vi "Replace a Substring.vi"() -> ()   [LabVIEW 2016]
panel:
  out "Replaced Sub-String":string
  out "Result String":string
  in  "Offset":dbl
  in  "Sub-String":string
  in  "String":string
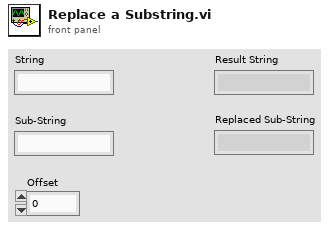
[diagram p1: front panel]
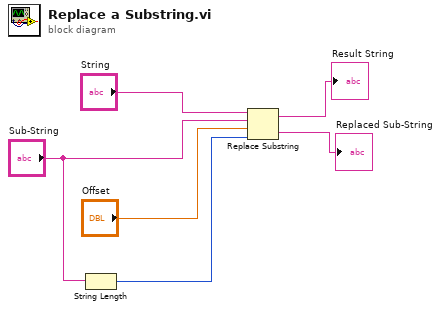
[diagram p0: block diagram]
diagram:
  n1 = String Length(string="Sub-String") -> (length=w2:i32)
  n2 = Replace Substring(2:w2, 3:"Offset", 4:"Sub-String", 5:"String") -> (0:→"Replaced Sub-String":string, 1:→"Result String":string)
